vi "Test PINGRESP packet.vi"(8 "error in (no error)":errorcluster) -> (0 "error out":errorcluster)   [LabVIEW 2013]
uses:
  source/Control Packets/PINGRESP/PINGRESP.lvclass
  source/Control Packets/ControlPacket/ControlPacket.lvclass/ControlPacket.ctl
  source/Control Packets/ControlPacket/ControlPacket.lvclass
panel:
  out "Packet ID":u16 format="%04x"
  out "Absence of Packet Identifier":bool
  out "Packet type":bool
  out "All packets consumed":bool
  out "Complete Packet":bool
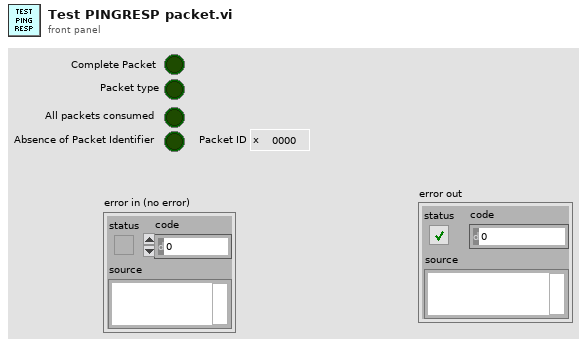
[diagram p1: front panel]
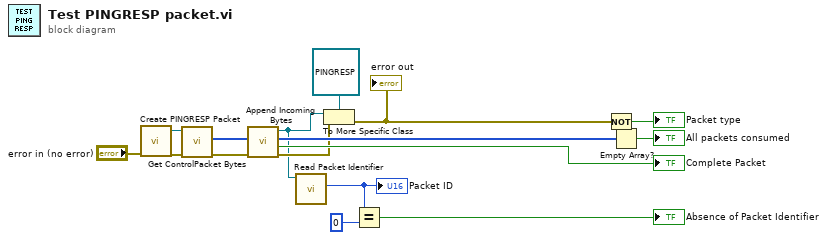
[diagram p0: block diagram]
diagram:
  n1 = call "Create PINGRESP Packet.vi"("error in (no error)"="error in (no error)") -> ("error out"=w3:errorcluster, "PINGRESP out"=w4:refnum<class "PINGRESP.lvclass">)  [unwired: 9 in]
  n2 = call "Get ControlPacket Bytes.vi"("error in (no error)"=w3, "ControlPacket"=w4) -> ("error out"=w10:errorcluster, "Bytes Stream"=w16:u8[])  [unwired: 6 in, 2 out]
  n3 = call "Append Incoming Bytes.vi"("error in (no error)"=w10, "Incoming Packets"=w16) -> ("error out"=w9:errorcluster, "Complete Packet"=→"Complete Packet":bool, "Remaining Packets"=w14:u8[], "ControlPacket"=w6:refnum<class "ControlPacket.lvclass">)  [unwired: 6 in]
  n4 = call "Read Packet Identifier.vi"("ControlPacket in"=w6) -> ("Packet Identifier"=w8:u16)  [unwired: 9 in, 1 out]
  "Packet ID" <- w8
  n5 = To More Specific Class(target class=refnum<class "PINGRESP.lvclass"> refnum ("MQTT_Control_Packets.lvlib:PINGRESP.lvclass"), reference=w6, error in=w9) -> (error out=w12:errorcluster)  [unwired: 1 out]
  "error out" <- w12
  n6 = Equal?(x=w8, y=u16 0) -> (x = y?=→"Absence of Packet Identifier":bool)
  n7 = Not(x=w12) -> (.not. x?=→"Packet type":bool)
  n8 = Empty Array?(array=w14) -> (empty?=→"All packets consumed":bool)
